vi "Bundle FPGA Configuration.vi"(8 "error in (no error)":errorcluster, 11 "FPGA VI Reference Out":refnum<k20>) -> (0 "error out":errorcluster, 3 "Cluster":T3)   [LabVIEW 2017]
uses:
  controls/FPGA State.ctl
  controls/Chatter data.ctl
  <vilib>/Utility/error.llb/Error Cluster From Error Code.vi
  <vilib>/rvi/errors/niLvFpgaAdjustHostInterfaceError.vi
  <vilib>/rvi/interface/nirviReadWriteControl/nirviReadWriteControl.xnode
  NiFpgaLv.dll
  <vilib>/rvi/interface/Simulation/niFpgaSimulationCallBeginRW.vi
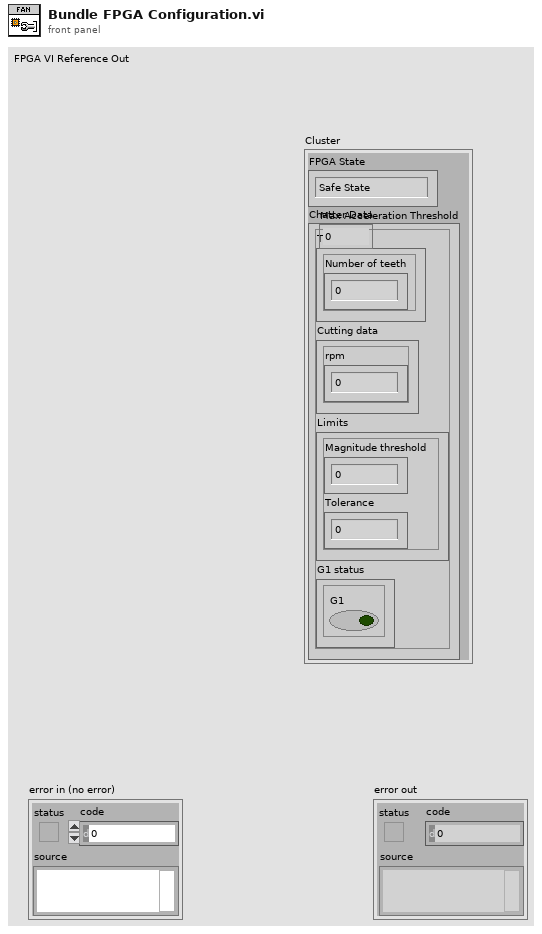
[diagram p1: front panel]
types:
  T1 = typedef "FPGA State.ctl" = enum16{"Safe State", "Control (PID)"}
  T2 = typedef "Chatter data.ctl" = cluster{"Tool data":cluster{"Number of teeth":sgl}, "Cutting data":cluster{"rpm":sgl}, "Limits":cluster{"Magnitude threshold":sgl, "Tolerance":sgl}, "G1 status":cluster{"G1 ":bool}}
  T3 = cluster{"FPGA State":T1, "Max Acceleration Threshold":sgl, "Chatter Data":T2}
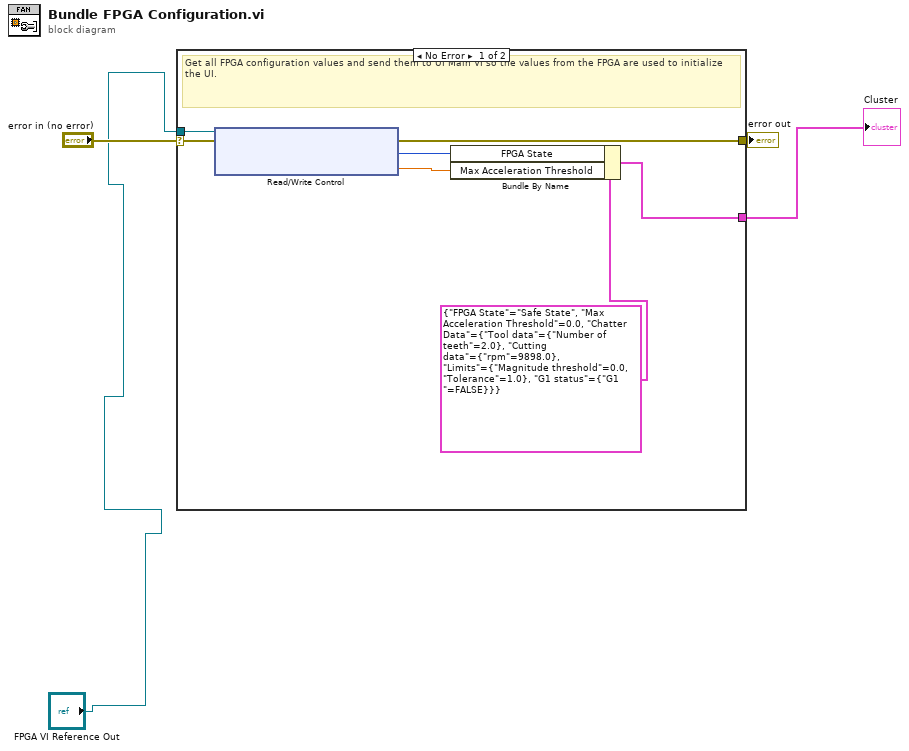
[diagram p0: block diagram]
diagram:
  n1 = case shown="No Error" "error in (no error)" {
    selector: "error in (no error)" -> [w11 w12]
    tunnel: "FPGA VI Reference Out" -> [w10 _]
    tunnel: [w9 w12] -> w3
    tunnel: [w8 _] -> w2
    frame No Error {
      # "Get all FPGA configuration values and send them to UI Main VI so the values from the FPGA are used to initialize the UI."
      n2 = xnode "Read/Write Control"("FPGA VI Reference In"=w10, "error in"=w11) -> ("error out"=w9:errorcluster, "Current FPGA State"=w7:enum16{"Safe State", "Control (PID)"}, "Max Acceleration Threshold (g)"=w6:sgl)  [unwired: 1 out]
      n3 = Bundle By Name(cluster=T3 {"FPGA State"=enum."Safe State", "Max Acceleration Threshold"=0.0, "Chatter Data"={"Tool data"={"Number of teeth"=2.0}, "Cutting data"={"rpm"=9898.0}, "Limits"={"Magnitude threshold"=0.0, "Tolerance"=1.0}, "G1 status"={"G1 "=FALSE}}}, "FPGA State"=w7, "Max Acceleration Threshold"=w6) -> (w8:T3)
    }
    frame Error {
      # "Error"
    }
  }
  "error out" <- w3
  "Cluster" <- w2
